vi "Simple Controls GUI.vi"() -> ()   [LabVIEW 2020]
panel:
  in  "String":string
  in  "Numeric":dbl
  in  "Button":bool
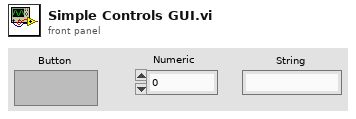
[diagram p1: front panel]
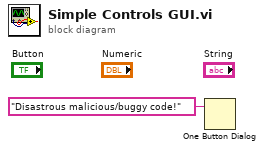
[diagram p0: block diagram]
diagram:
  n1 = One Button Dialog(message="Disastrous malicious/buggy code!") -> ()  [unwired: 1 in, 1 out]
